vi "Get 2D EXT.vi"(5 "format string (%_20f)":string="%_20f", 7 "key description":string, 8 "sections":string[](array[string]), 9 "numeric":ext[][](array[numeric]), 11 "info data":string) -> (0 "sections out":string[](array[string]), 2 "value":ext[][](array[numeric]) format="%.2f", 3 "info data out":string)   [LabVIEW 2019, in "infolib.lvlib"]
doc: "Add a new numeric key to Info Data string. If section exists in Info Data string, inserts key into this section."
uses:
  infolib.lvlib
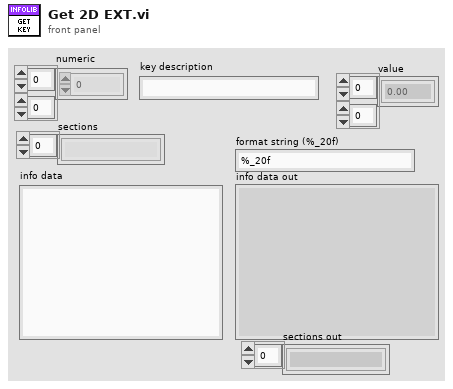
[diagram p1: front panel]
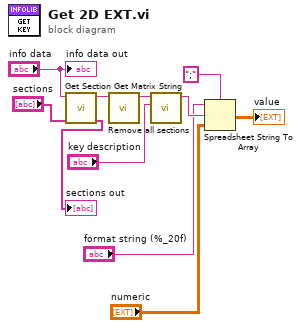
[diagram p0: block diagram]
diagram:
  n1 = call "Get Section.vi"("sections"="sections", "info data"="info data") -> ("sections out"=→"sections out":string[], "section part"=w11:string)  [unwired: 7 in, 1 out]
  n2 = call "Remove all sections.vi"("info data"=w11) -> ("info data out"=w9:string)  [unwired: 10 in]
  n3 = call "Get Matrix String.vi"("matrix key"="key description", "info data"=w9) -> ("matrix part"=w6:string)  [unwired: 8 in, 1 out]
  n4 = Spreadsheet String To Array(delimiter (Tab)=";", format string="format string (%_20f)", spreadsheet string=w6, array type (2D Dbl)="numeric") -> (array=→"value":ext[][])
  "info data out" <- "info data"
